vi "Write INIndex.vi"(8 "error in (no error)":errorcluster, 10 "INIndex":i32, 11 "Vision AI in":refnum<class "Vision AI.lvclass">) -> (0 "error out":errorcluster, 3 "Vision AI out":refnum<class "Vision AI.lvclass">)   [LabVIEW 2019, in "Vision AI.lvclass"]
uses:
  Vision AI.lvclass
  FlowIOCtrl.lvclass
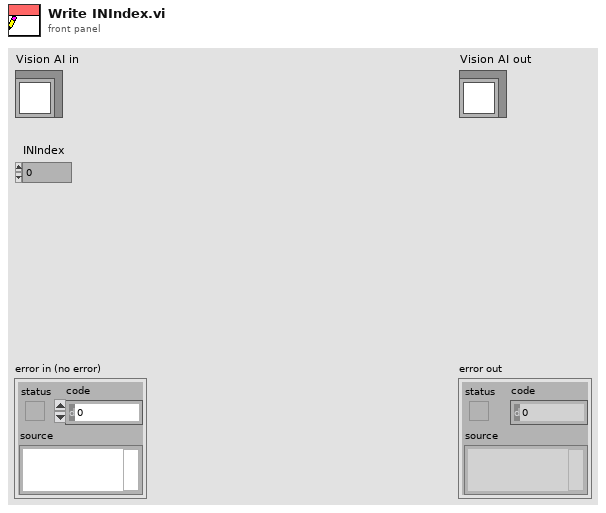
[diagram p1: front panel]
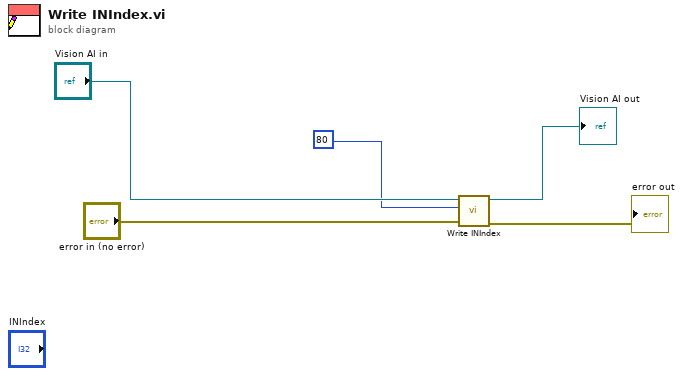
[diagram p0: block diagram]
diagram:
  n1 = call-parent "Write INIndex.vi"("error in (no error)"="error in (no error)", "INIndex"=80, "Station Action in"="Vision AI in") -> ("error out"=→"error out":errorcluster, "Station Action out"=→"Vision AI out":refnum<class "Vision AI.lvclass">)  [unwired: 7 in]
